vi "mod_Create Continuous PSK.vi"(0 "PN Sequence Order":i32, 1 "Symbol Rate, Hz":dbl format="%.2f", 2 "Custom-PSK Parameters":T1 {"PSK type" items=["normal", "shifted", "offset"]; "symbol map" format="%.3f"}, 3 "TX Filter":T2(ring), 4 "Filter Length":i32, 5 "Alpha":dbl format="%.2f") -> (6 "samples per symbol":i32, 7 "output complex waveform":T3 {"Y" format="%.3f"; "dt" format="%^.2e"; "t0" format="%.4f"}, 8 "error out":errorcluster)   [LabVIEW 2020, in "niDMT.lvlib"]
uses:
  <vilib>/addons/Modulation/niDMT.lvlib
  <vilib>/addons/Modulation/Analog/controls/Complex Data Waveform.ctl
  <vilib>/addons/Modulation/Digital/Support/Controls/PSK System Parameters.ctl
  <vilib>/addons/Modulation/Analog/support/mod_Set Error Source.vi
  <vilib>/addons/Modulation/Digital/Support/Common/Validators/mod_Generate Bits Validate.vi
  <vilib>/addons/Modulation/Digital/General/subVIs/mod_Generate Bits Pattern.vi
  <vilib>/addons/Modulation/Digital/Support/Common/Validators/mod_Generate Filter Coefficients Validate.vi
  <vilib>/addons/Modulation/Digital/General/subVIs/mod_Generate Filter Coefficients.vi
  <vilib>/addons/Modulation/Digital/General/subVIs/mod_Generate Bits PN Sequence.vi
  <vilib>/addons/Modulation/niAMT.lvlib
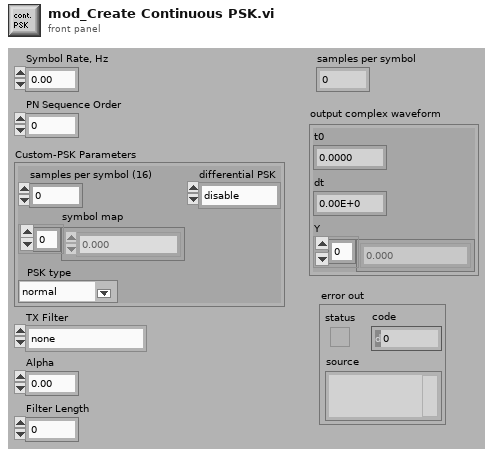
[diagram p1: front panel]
types:
  T1 = typedef "niDMT.lvlib/PSK System Parameters.ctl" = cluster{"samples per symbol (16)":i32, "symbol map":cdb[], "differential PSK":enum16{"disable", "enable"}, "PSK type":u16}
  T2 = enum16{"none", "Raised Cosine", "Root Raised Cos", "Gaussian"}
  T3 = typedef "niAMT.lvlib/Complex Data Waveform.ctl" = cluster{"t0":dbl, "dt":dbl, "Y":cdb[]}
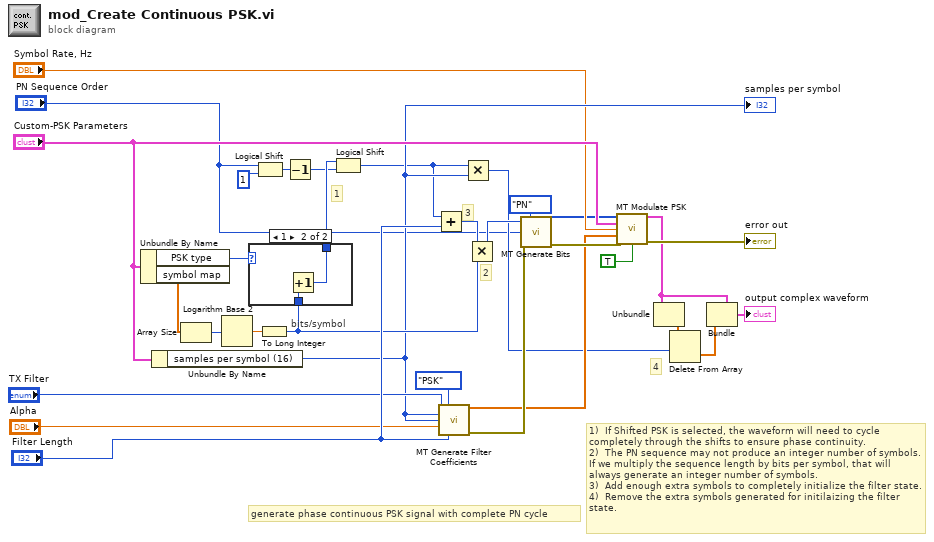
[diagram p0: block diagram]
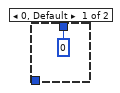
[diagram p2: hidden frame]
diagram:
  # "4"
  # "2"
  # "1"
  # "3"
  # "1)  If Shifted PSK is selected, the waveform will need to cycle completely through the shifts to ensure phase continuity. \n2)  The PN sequence may not produce an integer number of symbols.  If we multiply the sequence length by bits per symbol, that will always generate an integer number of symbols. \n3)  Add enough extra symbols to completely initialize the filter state.\n4)  Remove the extra symbols generated for initilaizing the filter state."
  # "bits/symbol"
  # "generate phase continuous PSK signal with complete PN cycle"
  n1 = Unbundle By Name("Custom-PSK Parameters") -> ("PSK type"=w1:u16, "symbol map"=w6:cdb[])
  n2 = Unbundle By Name("Custom-PSK Parameters") -> ("samples per symbol (16)"=w21:i32)
  "samples per symbol" <- w21
  n3 = Array Size(array=w6) -> (size(s)=w8:i32)
  n4 = Logarithm Base 2(1:w8) -> (0:w9:dbl)
  n5 = Logical Shift(y="PN Sequence Order", x=1) -> (x << y=w5:i32)
  n6 = To Long Integer(number=w9) -> (32bit integer=w22:i32)
  n7 = case shown="1" w1 {
    tunnel: w22 -> [_ w35]
    tunnel: [0 w34] -> w13
    frame 0, Default {
    }
    frame 1 {
      n8 = Increment(x=w35) -> (x+1=w34:i32)
    }
  }
  n9 = Decrement(x=w5) -> (x-1=w12:i32)
  n10 = Logical Shift(y=w13, x=w12) -> (x << y=w7:i32)
  n11 = Add(x=w7, y="Filter Length") -> (x+y=w23:i32)
  n12 = call <vilib>:"MT Generate Filter Coefficients.vi"("pulse shaping filter (none)"="TX Filter", "modulation type"=enum16{"FSK", "PSK", "QAM", "MSK"}."PSK" ("Modulation Type"), "pulse shaping samples per symbol (16)"=w21, "matched samples per symbol (16)"=w21, "filter parameter"="Alpha", "filter length (symbols)"="Filter Length") -> ("pulse shaping filter coefficients"=w16:dbl[], "error out"=w26:errorcluster)  [unwired: 1 in, 7 out]
  n13 = Multiply(x=w7, y=w21) -> (x*y=w14:i32)
  n14 = Multiply(x=w23, y=w22) -> (x*y=w24:i32)
  n15 = call <vilib>:"MT Generate Bits.vi"("total bits (128)"=w24, "mode (PN)"=enum16{"PN", "pattern", "user"}."PN" ("Mode (PN)"), "PN sequence order (9)"="PN Sequence Order", "error in (no error)"=w26) -> ("output bit stream"=w15:i8[], "error out"=w27:errorcluster)  [unwired: 4 in, 6 out]
  n16 = call <vilib>:"MT Modulate PSK.vi"("input bit stream"=w15, "PSK system parameters"="Custom-PSK Parameters", "symbol rate (Hz)"="Symbol Rate, Hz", "pulse shaping filter coefficients"=w16, "error in (no error)"=w27, "reset? (T)"=TRUE ("Reset (T)")) -> ("output complex waveform"=w18:T3, "error out"=→"error out":errorcluster)  [unwired: 1 in, 7 out]
  n17 = Unbundle(w18) -> ("Y"=w10:cdb[])  [unwired: 2 out]
  n18 = Delete From Array(array=w10, length=w14) -> (deleted portion=w11:cdb[])  [unwired: 1 in, 1 out]
  n19 = Bundle(cluster=w18, "Y"=w11) -> (→"output complex waveform":T3)  [unwired: 2 out]
